vi "Set Multi.vi"(0 "Display State In":T2, 5 "Value In":T1, 7 "First?":bool, 9 "Container State":T3, 11 "error in (no error)":errorcluster) -> (4 "Display State Out":T2, 15 "error out":errorcluster)   [LabVIEW 2015, in "Tone (G3).xctl"]
uses:
  Tone (G3).xctl
  <vilib>/_xctls/Container State.ctl
  State.ctl
  Utility VIs/Controls/KNumeric (DBL)/KNumeric (DBL).xctl
  Utility VIs/Controls/KCheckbox/KCheckbox.xctl
  Tone.Properties.ctl
  <vilib>/_xctls/XControlSupport.lvlib
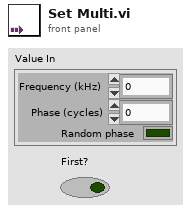
[diagram p1: front panel]
types:
  T1 = typedef "Tone (G3).xctl/Tone.Properties.ctl" = cluster{"Frequency (kHz)":dbl, "Phase (cycles)":dbl, "Random phase":bool}
  T2 = typedef "Tone (G3).xctl/State.ctl" = cluster{"enable menu":bool, "ctls":cluster{"Freq":refnum<vi>, "Phase":refnum<vi>, "Random":refnum<vi>}}
  T3 = typedef "XControlSupport.lvlib/Container State.ctl" = cluster{"Indicator?":bool, "Run Mode?":bool, " Refnum":refnum<vi>}
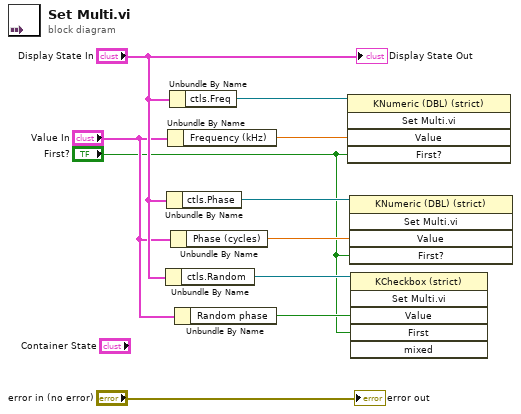
[diagram p0: block diagram]
diagram:
  n1 = Unbundle By Name("Display State In") -> ("ctls.Random"=w5:refnum<vi>)
  n2 = Unbundle By Name("Display State In") -> ("ctls.Phase"=w8:refnum<vi>)
  n3 = Unbundle By Name("Value In") -> ("Frequency (kHz)"=w1:dbl)
  n4 = Unbundle By Name("Display State In") -> ("ctls.Freq"=w9:refnum<vi>)
  n5 = Unbundle By Name("Value In") -> ("Phase (cycles)"=w7:dbl)
  n6 = Unbundle By Name("Value In") -> ("Random phase"=w3:bool)
  n7 = invoke class="KNumeric (DBL) (strict)" method="Set Multi.vi"(reference=w9, "Value"=w1, "First?"="First?") -> ()  [unwired: 2 in, 5 out]
  n8 = invoke class="KNumeric (DBL) (strict)" method="Set Multi.vi"(reference=w8, "Value"=w7, "First?"="First?") -> ()  [unwired: 2 in, 5 out]
  n9 = invoke class="KCheckbox (strict)" method="Set Multi.vi"(reference=w5, "Value"=w3, "First"="First?") -> ()  [unwired: 3 in, 6 out]
  "Display State Out" <- "Display State In"
  "error out" <- "error in (no error)"
